vi "interrupt routine.vi"(8 "error in (no error)":errorcluster, 11 "Template in":refnum<class "Template.lvclass">) -> (0 "error out":errorcluster, 3 "Template out":refnum<class "Template.lvclass">)   [LabVIEW 2020, in "Template.lvlib" / "Template.lvclass"]
doc: "Executes the interrupt routine in the defined timeout intervals as per the ActorConfiguration.\nThis is called in the \"loop helper.vi\" executed in the Actor Core.vi override"
uses:
  Template.lvclass
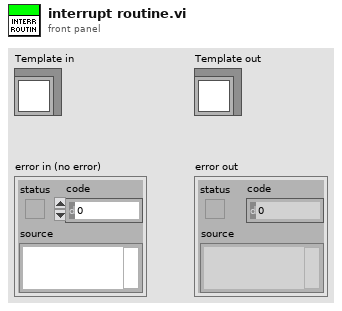
[diagram p1: front panel]
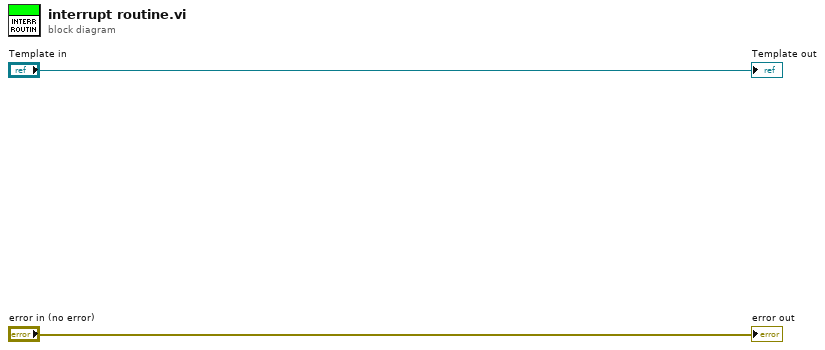
[diagram p0: block diagram]
diagram:
  "error out" <- "error in (no error)"
  "Template out" <- "Template in"
